vi "DriveForTime-C.vi"(11 "Params":string[][](array[string])) -> ()   [LabVIEW 2017]
uses:
  Framework/Robot Global Data.vi
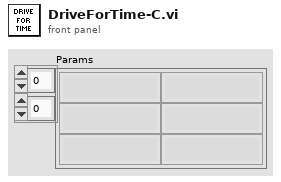
[diagram p1: front panel]
types:
  T1 = typedef "Command Status Info.ctl" = cluster{"Name":string, "Status":T2, "notifier out":T3}
  T2 = typedef "Completion Status.ctl" = enum16{"Successful", "Aborted", "Incomplete"}
  T3 = typedef "Completion Notifier.ctl" = refnum<notifier>
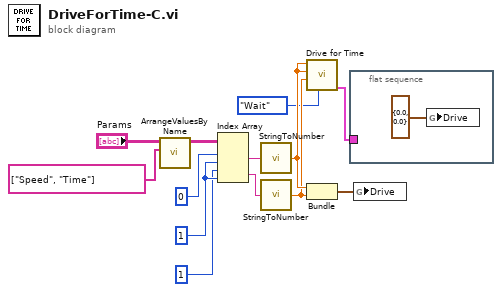
[diagram p0: block diagram]
diagram:
  w5 = 1
  n1 = call "ArrangeValuesByName.vi"("Names"=string[] ["Speed", "Time"], "Names/Values in"="Params") -> ("Names/Values Out"=w7:string[][])  [unwired: 9 in]
  n2 = Index Array(array=w7, index (row) #1=0, index (col) #1=w5, index (row) #2=1, index (col) #2=w5) -> (element #1=w3:string, element #2=w1:string)
  n3 = call "StringToNumber.vi"("String"=w3) -> ("Output"=w12:dbl)
  n4 = call "StringToNumber.vi"("String"=w1) -> ("Output"=w11:dbl)
  n5 = call "Drive for Time.vi"("Synchronization"=enum16{"Start", "Wait"}."Wait", "Seconds"=w11, "Right Speed"=w12, "Left Speed"=w12) -> ("Command Info Out"=w9:T1)  [unwired: 6 in, 1 out]
  n6 = Bundle("Output"=w12, "Output"=w11) -> (w13:cluster{"Output":dbl, "Output":dbl})  [unwired: 1 in]
  n7 = flat-sequence {
    tunnel: w9 -> [_]
    frame #0 {
      n8 = global write "Robot Global Data.vi" "Drive"(cluster{"Drive Speed":dbl, "Drive Time":dbl} {"Drive Speed"=0.0, "Drive Time"=0.0} ("Drive")) -> ()
    }
  }
  n9 = global write "Robot Global Data.vi" "Drive"(w13) -> ()
